vi "Control Panel Teleop.vi"   [LabVIEW 2019]
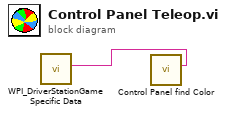
[diagram p0: block diagram]
diagram:
  n1 = call <vilib>:"WPI_DriverStationGame Specific Data.vi"() -> ("Game Specific Data"=w1:string)  [unwired: 11 in]
  n2 = call "Control Panel find Color.vi"("Expected Color"=w1) -> ()  [unwired: 9 in, 1 out]
